vi "Calculate_error.vi"(0 "x 2":dbl, 1 "x 1":dbl, 2 "Button":bool, 3 "file path (dialog if empty)":path) -> (4 "Calibration Curve":cluster{"Best Linear Fit":dbl[], dbl[]}[](graph), 5 "Calibration parameters":T1, 6 "Slide":u8(slide) scale=0.0..100.0)   [LabVIEW 2018]
uses:
  <vilib>/Analysis/5stat.llb/RMS (DBL).vi
  <vilib>/Utility/file.llb/Write Delimited Spreadsheet (DBL).vi
  <vilib>/Analysis/NI_AALPro.lvlib
  <vilib>/ptbypt/NI_PtbyPt.lvlib
  <vilib>/Analysis/NI_AALBase.lvlib
panel:
  in  "x 4":dbl[](array[numeric])
  in  "x 3":dbl[](array[numeric])
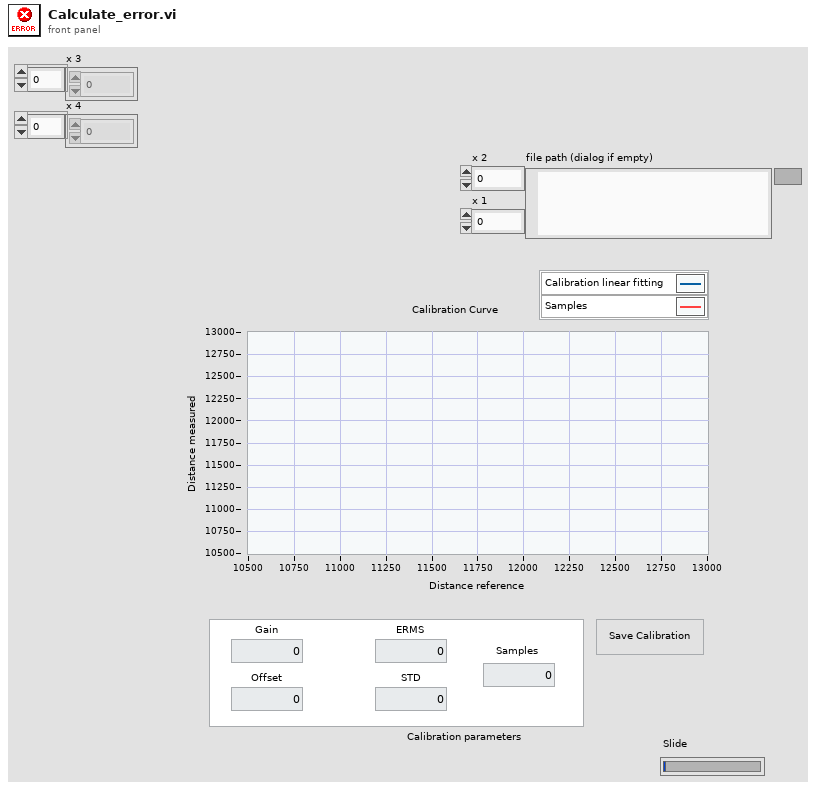
[diagram p1: front panel]
types:
  T1 = cluster{"Gain":dbl, "Offset":dbl, "ERMS":dbl, "STD":dbl, "Samples ":dbl}
  T2 = cluster{"slope":dbl, "intercept":dbl, dbl, dbl, i32}
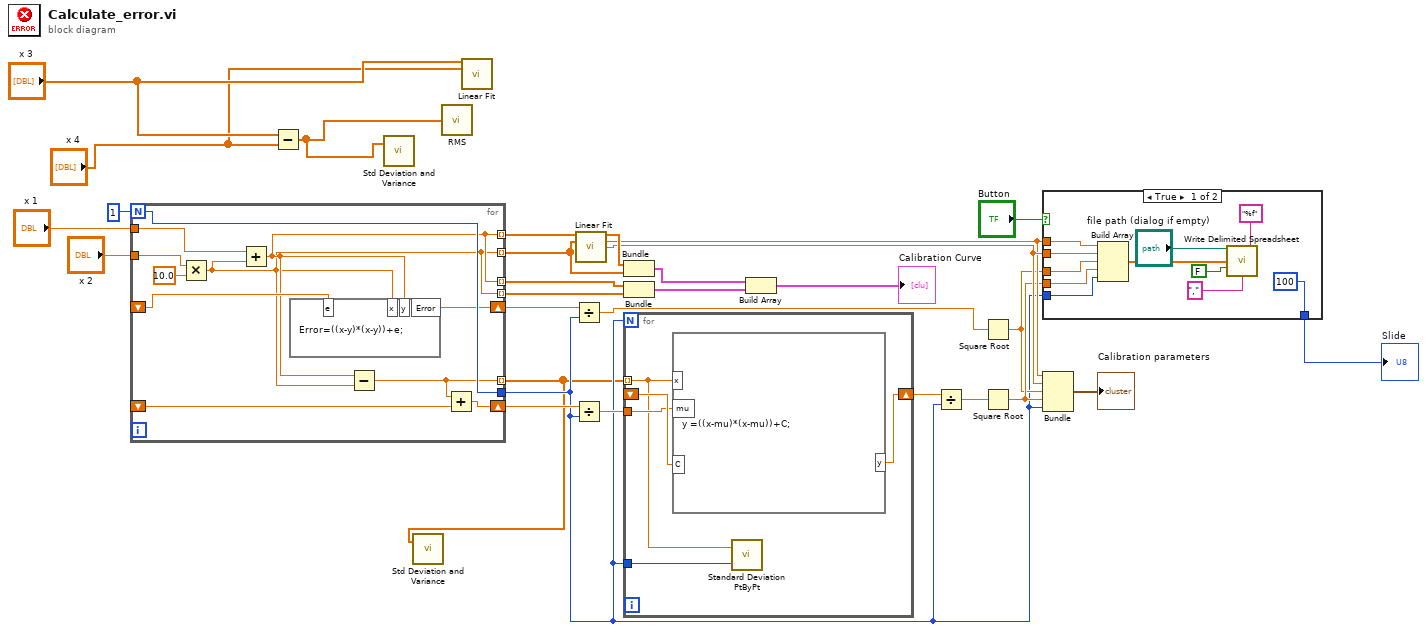
[diagram p0: block diagram]
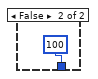
[diagram p2: hidden frame]
diagram:
  n1 = for {
    N: 1 -> [w40]
    tunnel: [w33] -> w19 mode=indexing
    tunnel: [w32] -> w18 mode=indexing
    tunnel: [w33] -> w26 mode=indexing
    tunnel: [w32] -> w25 mode=indexing
    shift-right: [w39] -> w17
    shift-left: _ -> [w37]
    tunnel: [w40] -> w5
    tunnel: [w38] -> w4 mode=indexing
    shift-right: [w36] -> w15
    shift-left: _ -> [w35]
    tunnel: "x 2" -> [w31]
    tunnel: "x 1" -> [w30]
    n2 = Multiply(x=w31, y=10.0) -> (x*y=w32:dbl)
    n3 = Add(x=w30, y=w32) -> (x+y=w33:dbl)
    n4 = formula code="Error=((x-y)*(x-y))+e;"("x"=w32, "y"=w33, "e"=w37) -> ("Error"=w39:dbl)
    n5 = Subtract(x=w33, y=w32) -> (x-y=w38:dbl)
    n6 = Add(x=w38, y=w35) -> (x+y=w36:dbl)
  }
  n7 = Subtract(x="x 3", y="x 4") -> (x-y=w1:dbl[])
  n8 = call <vilib>:"Std Deviation and Variance.vi"("X"=w1) -> ()  [unwired: 1 in, 3 out]
  n9 = call <vilib>:"Std Deviation and Variance.vi"("X"=w4) -> ()  [unwired: 1 in, 3 out]
  n10 = call-poly <vilib>:"RMS.vi"("X"=w1) -> ()  [unwired: 2 out]
  n11 = call <vilib>:"Linear Fit.vi"("Y"="x 3", "X"="x 4") -> ()  [unwired: 9 in, 5 out]
  n12 = Divide(x=w17, y=w5) -> (x/y=w16:dbl)
  n13 = Divide(x=w15, y=w5) -> (x/y=w10:dbl)
  n14 = call <vilib>:"Linear Fit.vi"("Y"=w19, "X"=w18) -> ("Best Linear Fit"=w28:dbl[], "slope"=w20:dbl, "intercept"=w21:dbl)  [unwired: 9 in, 2 out]
  n15 = Bundle("Best Linear Fit"=w28, w18) -> (w27:cluster{"Best Linear Fit":dbl[], dbl[]})  [unwired: 1 in]
  n16 = Bundle(w26, w25) -> (w24:cluster{dbl[], dbl[]})  [unwired: 1 in]
  n17 = for {
    N: w5 -> [_]
    shift-right: [w44] -> w9
    shift-left: _ -> [w45]
    tunnel: w10 -> [w43]
    tunnel: w4 -> [w42] mode=indexing
    tunnel: w5 -> [w41]
    n18 = formula code="y =((x-mu)*(x-mu))+C;"("x"=w42, "C"=w45, "mu"=w43) -> ("y"=w44:dbl)
    n19 = call <vilib>:"Standard Deviation PtByPt.vi"("x"=w42, "sample length"=w41) -> ()  [unwired: 1 in, 3 out]
  }
  n20 = Build Array(w27, w24) -> (→"Calibration Curve":cluster{"Best Linear Fit":dbl[], dbl[]}[])
  n21 = Divide(x=w9, y=w5) -> (x/y=w14:dbl)
  n22 = Square Root(x=w16) -> (sqrt(x)=w11:dbl)
  n23 = Square Root(x=w14) -> (sqrt(x)=w12:dbl)
  n24 = case shown="True" "Button" {
    tunnel: w21 -> [w52 _]
    tunnel: w20 -> [w51 _]
    tunnel: w5 -> [w50 _]
    tunnel: w12 -> [w48 _]
    tunnel: w11 -> [w49 _]
    tunnel: [u8 100 ("Slide") u8 100 ("Slide")] -> w6
    frame True {
      n25 = Build Array(w51, w52, w49, w48, w50) -> (w56:dbl[])
      n26 = call-poly <vilib>:"Write Delimited Spreadsheet.vi"("file path (dialog if empty)"="file path (dialog if empty)", "format (%.3f)"="%f", "1D data"=w56, "append to file? (new file:F)"=FALSE, "delimiter (\\t)"="," ("delimiter (\\t)")) -> ()  [unwired: 9 in, 2 out]
    }
    frame False {
    }
  }
  "Slide" <- w6
  n27 = Bundle("slope"=w20, "intercept"=w21, w11, w12, w5) -> (→"Calibration parameters":T2)  [unwired: 1 in]
